vi "Signal_measurements_test.vi"(8 "error in (no error)":errorcluster, 11 "Input waveform":waveform(dbl)) -> (0 "error out":errorcluster, 1 "Measured frequency":dbl, 2 "Measured amplitude":dbl, 3 "String":string)   [LabVIEW 2019]
uses:
  <vilib>/measure/madcrms.llb/Basic Averaged DC-RMS for 1 Chan.vi
  <vilib>/measure/NI_MAPro.lvlib
  <vilib>/measure/mascope.llb/Transition Measurements 1 chan.vi
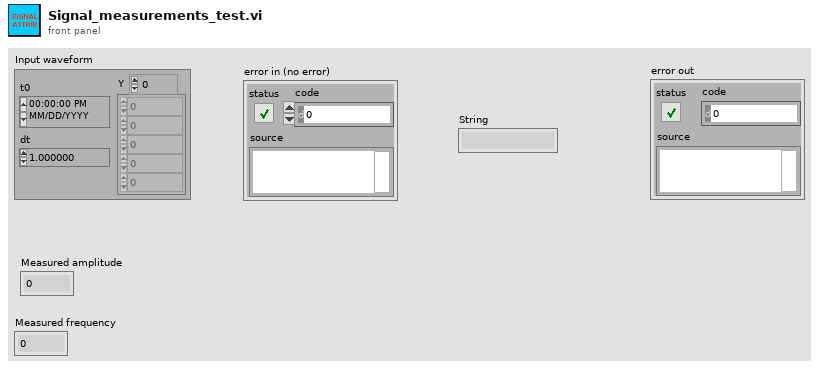
[diagram p1: front panel]
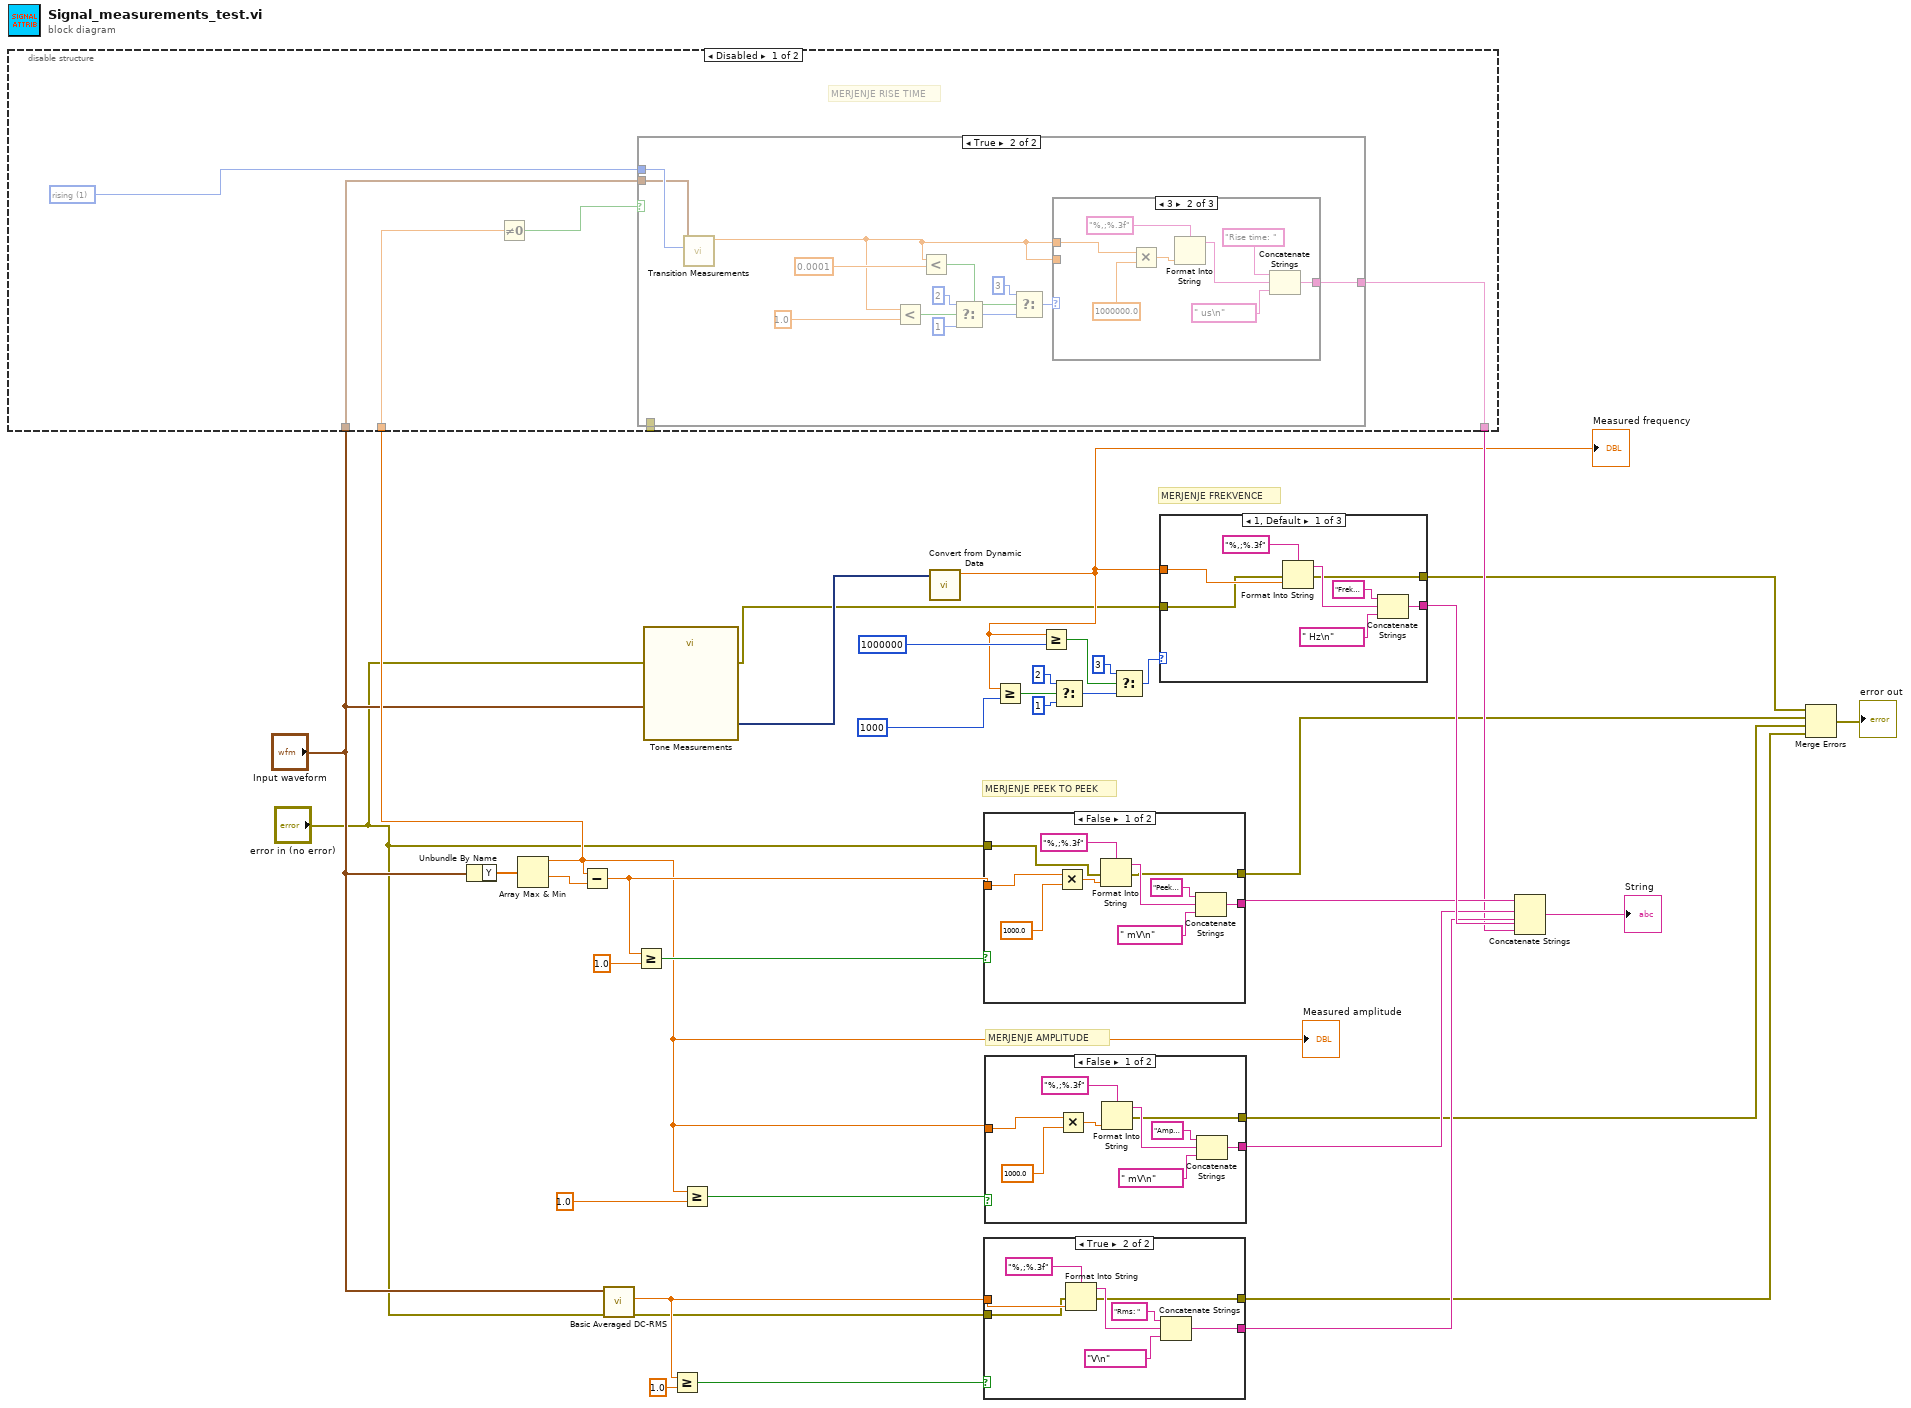
[diagram p0: block diagram]
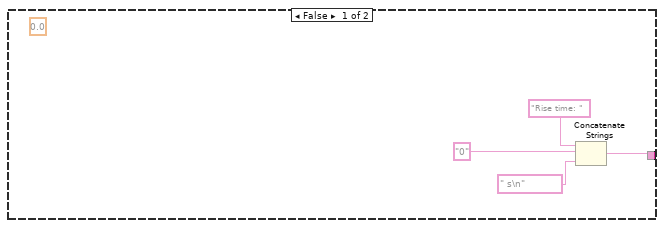
[diagram p2: hidden frame]
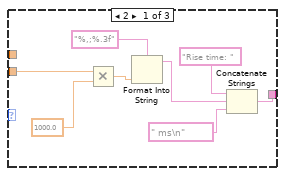
[diagram p3: hidden frame]
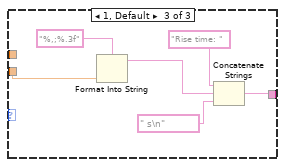
[diagram p4: hidden frame]
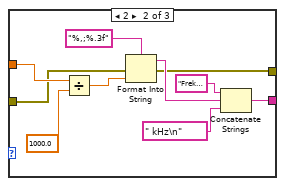
[diagram p6: hidden frame]
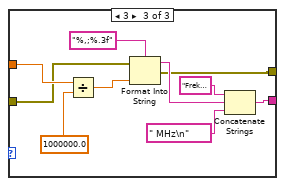
[diagram p7: hidden frame]
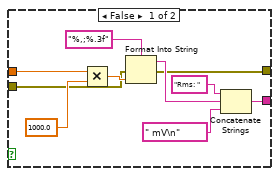
[diagram p8: hidden frame]
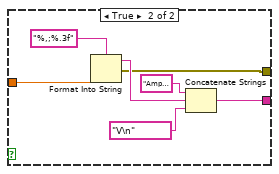
[diagram p9: hidden frame]
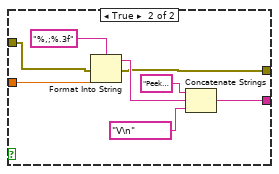
[diagram p10: hidden frame]
diagram:
  # "MERJENJE FREKVENCE"
  # "MERJENJE AMPLITUDE"
  # "MERJENJE PEEK TO PEEK"
  n1 = Unbundle By Name("Input waveform") -> ("Y"=w34:dbl[])
  n2 = Array Max & Min(array=w34) -> (max value=w22:dbl, min value=w23:dbl)  [unwired: 2 out]
  "Measured amplitude" <- w22
  n3 = disable-structure shown="Disabled" {
    disable-tunnel: "Input waveform" -> [w42 _]
    disable-tunnel: _ -> [w41 _]
    disable-tunnel: w22 -> [w40 _]
    disable-tunnel: [w38 _] -> w12
    frame Disabled {
      w43 = u16 1 items=["falling", "rising"] ("polarity (rising)")
      # "MERJENJE RISE TIME"
      n4 = Not Equal To 0?(x=w40) -> (x != 0?=w39:bool)
      n5 = case shown="True" w39 {
        tunnel: w43 -> [_ w60]
        tunnel: w42 -> [_ w59]
        tunnel: w41 -> [_ _]
        tunnel: [w45 w49] -> w38
        frame False {
          (unwired) 0.0 ("transition duration")
          n6 = Concatenate Strings("Rise time: " ("string"), "0" ("string"), " s\n") -> (w45:string)
        }
        frame True {
          n7 = call-poly <vilib>:"Transition Measurements.vi"("polarity (rising)"=w60, "signal in"=w59) -> ("transition duration"=w48:dbl)  [unwired: 4 in, 5 out]
          n8 = Less?(x=w48, y=1.0) -> (x < y?=w58:bool)
          n9 = Less?(x=w48, y=0.0001) -> (x < y?=w56:bool)
          n10 = Select(t=2, s=w58, f=1 ("t")) -> (s? t:f=w57:i32)
          n11 = Select(t=3, s=w56, f=w57) -> (s? t:f=w50:i32)
          n12 = case shown="3" w50 {
            tunnel: [w63 w70 w80] -> w49
            tunnel: w48 -> [_ w69 _]
            tunnel: w48 -> [w61 _ w77]
            frame 2 {
              n13 = Multiply(x=w61, y=1000.0) -> (x*y=w64:dbl)
              n14 = Format Into String(format string="%,;%.3f", w64) -> (resulting string=w67:string)  [unwired: 2 in, 1 out]
              n15 = Concatenate Strings("Rise time: " ("string"), w67, " ms\n") -> (w63:string)
            }
            frame 3 {
              n16 = Multiply(x=w69, y=1000000.0) -> (x*y=w72:dbl)
              n17 = Format Into String(format string="%,;%.3f", w72) -> (resulting string=w75:string)  [unwired: 2 in, 1 out]
              n18 = Concatenate Strings("Rise time: " ("string"), w75, " us\n") -> (w70:string)
            }
            frame 1, Default {
              n19 = Format Into String(format string="%,;%.3f", w77) -> (resulting string=w79:string)  [unwired: 2 in, 1 out]
              n20 = Concatenate Strings("Rise time: " ("string"), w79, " s\n") -> (w80:string)
            }
          }
        }
      }
    }
    frame Enabled {
    }
  }
  n21 = Subtract(x=w22, y=w23) -> (x-y=w26:dbl)
  n22 = call-poly <vilib>:"Basic Averaged DC-RMS.vi"("error in (no error)"="error in (no error)", "signal in"="Input waveform") -> ("error out"=w2:errorcluster, "RMS value"=w36:dbl)  [unwired: 6 in, 2 out]
  n23 = Greater Or Equal?(x=w26, y=1.0) -> (x >= y?=w24:bool)
  n24 = call "Tone Measurements"("error in (no error)"="error in (no error)", "Signals"="Input waveform") -> ("error out"=w7:errorcluster, "Frequency"=w10:dynamicdata)  [unwired: 8 in]
  n25 = Greater Or Equal?(x=w36, y=1.0) -> (x >= y?=w32:bool)
  n26 = Greater Or Equal?(x=w22, y=1.0) -> (x >= y?=w28:bool)
  n27 = call "Convert from Dynamic Data"("Dynamic Data Type"=w10) -> ("Scalar"=w9:dbl)  [unwired: 3 in]
  "Measured frequency" <- w9
  n28 = case shown="False" w24 {
    tunnel: [w85 w96] -> w30
    tunnel: w26 -> [w92 w95]
    tunnel: "error in (no error)" -> [w84 w94]
    tunnel: [w83 w93] -> w4
    frame False {
      n29 = Multiply(x=w92, y=1000.0) -> (x*y=w86:dbl)
      n30 = Format Into String(format string="%,;%.3f", error in=w84, w86) -> (resulting string=w90:string, error out=w83:errorcluster)  [unwired: 1 in]
      n31 = Concatenate Strings("Peek to peek: ", w90, " mV\n") -> (w85:string)
    }
    frame True {
      n32 = Format Into String(format string="%,;%.3f", error in=w94, w95) -> (resulting string=w100:string, error out=w93:errorcluster)  [unwired: 1 in]
      n33 = Concatenate Strings("Peek to peek: ", w100, "V\n") -> (w96:string)
    }
  }
  n34 = case shown="True" w32 {
    tunnel: [w104 w114] -> w33
    tunnel: w36 -> [w103 w113]
    tunnel: w2 -> [w102 w112]
    tunnel: [w101 w111] -> w1
    frame False {
      n35 = Multiply(x=w103, y=1000.0) -> (x*y=w105:dbl)
      n36 = Format Into String(format string="%,;%.3f", error in=w102, w105) -> (resulting string=w109:string, error out=w101:errorcluster)  [unwired: 1 in]
      n37 = Concatenate Strings("Rms: ", w109, " mV\n") -> (w104:string)
    }
    frame True {
      n38 = Format Into String(format string="%,;%.3f", error in=w112, w113) -> (resulting string=w118:string, error out=w111:errorcluster)  [unwired: 1 in]
      n39 = Concatenate Strings("Rms: ", w118, "V\n") -> (w114:string)
    }
  }
  n40 = case shown="False" w28 {
    tunnel: [w120 w130] -> w31
    tunnel: w22 -> [w127 w129]
    tunnel: [w119 w128] -> w3
    frame False {
      n41 = Multiply(x=w127, y=1000.0) -> (x*y=w121:dbl)
      n42 = Format Into String(format string="%,;%.3f", w121) -> (resulting string=w125:string, error out=w119:errorcluster)  [unwired: 2 in]
      n43 = Concatenate Strings("Amplituda:", w125, " mV\n") -> (w120:string)
    }
    frame True {
      n44 = Format Into String(format string="%,;%.3f", w129) -> (resulting string=w134:string, error out=w128:errorcluster)  [unwired: 2 in]
      n45 = Concatenate Strings("Amplituda: ", w134, "V\n") -> (w130:string)
    }
  }
  n46 = Greater Or Equal?(x=w9, y=1000) -> (x >= y?=w14:bool)
  n47 = Greater Or Equal?(x=w9, y=1000000) -> (x >= y?=w18:bool)
  n48 = Select(t=2, s=w14, f=1 ("t")) -> (s? t:f=w13:i32)
  n49 = Select(t=3, s=w18, f=w13) -> (s? t:f=w21:i32)
  n50 = case shown="1, Default" w21 {
    tunnel: [w138 w148 w156] -> w35
    tunnel: w9 -> [w137 w145 w155]
    tunnel: w7 -> [w136 w144 w154]
    tunnel: [w135 w143 w153] -> w5
    frame 1, Default {
      n51 = Format Into String(format string="%,;%.3f", error in=w136, w137) -> (resulting string=w142:string, error out=w135:errorcluster)  [unwired: 1 in]
      n52 = Concatenate Strings("Frekvenca: ", w142, " Hz\n") -> (w138:string)
    }
    frame 2 {
      n53 = Divide(x=w145, y=1000.0) -> (x/y=w147:dbl)
      n54 = Format Into String(format string="%,;%.3f", error in=w144, w147) -> (resulting string=w152:string, error out=w143:errorcluster)  [unwired: 1 in]
      n55 = Concatenate Strings("Frekvenca: ", w152, " kHz\n") -> (w148:string)
    }
    frame 3 {
      n56 = Divide(x=w155, y=1000000.0) -> (x/y=w162:dbl)
      n57 = Format Into String(format string="%,;%.3f", error in=w154, w162) -> (resulting string=w161:string, error out=w153:errorcluster)  [unwired: 1 in]
      n58 = Concatenate Strings("Frekvenca: ", w161, " MHz\n") -> (w156:string)
    }
  }
  n59 = Concatenate Strings(w30, w31, w33, w35, w12) -> (→"String":string)
  n60 = Merge Errors(w5, w4, w3, w1) -> (→"error out":errorcluster)
